vi "Получение данных.vi"(8 "error in (no error)":errorcluster, 11 "VISA Refnum in":refnum<visa-resource-name>) -> (0 "error out":errorcluster, 2 "String":string, 3 "VISA Refnum out":refnum<visa-resource-name>)   [LabVIEW 2013]
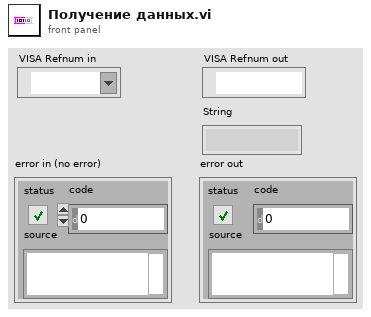
[diagram p1: front panel]
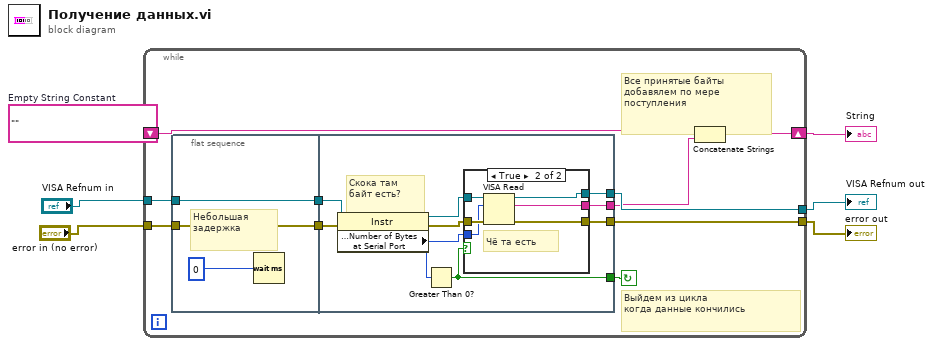
[diagram p0: block diagram]
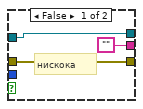
[diagram p2: hidden frame]
diagram:
  w1 = ""  # Empty String Constant
  n1 = while {
    tunnel: "VISA Refnum in" -> [w14]
    tunnel: "error in (no error)" -> [w13]
    tunnel: [w11] -> w2
    shift-right: [w8] -> w4
    shift-left: w1 -> [w10]
    tunnel: [w7] -> w3
    stop <- w12 continue-if-true
    # "Все принятые байты\nдобавялем по мере\nпоступления"
    # "Выйдем из цикла\nкогда данные кончились"
    n2 = flat-sequence {
      tunnel: w14 -> [w19]
      tunnel: w13 -> [w18]
      tunnel: [w19] -> w16
      tunnel: [w18] -> w15
      tunnel: w16 -> [w28]
      tunnel: w15 -> [w27]
      tunnel: [w23] -> w12
      tunnel: [w22] -> w9
      tunnel: [w21] -> w11
      tunnel: [w20] -> w7
      frame #0 {
        # "Небольшая\nзадержка"
        n3 = Wait (ms)(milliseconds to wait=u32 0) -> ()  [unwired: 1 out]
      }
      frame #1 {
        # "Скока там\nбайт есть?"
        n4 = property class="Instr"(reference=w28, error in=w27) -> (reference out=w26:refnum<visa-resource-name>, error out=w25:errorcluster, "Serial Settings:Number of Bytes at Serial Port"=w24:u32)
        n5 = Greater Than 0?(x=w24) -> (x > 0?=w23:bool)
        n6 = case shown="True" w23 {
          tunnel: w26 -> [w30 w37]
          tunnel: w25 -> [w31 w36]
          tunnel: w24 -> [_ w35]
          tunnel: [w31 w34] -> w20
          tunnel: [w30 w33] -> w21
          tunnel: ["" w32] -> w22
          frame False {
            # "нискока"
          }
          frame True {
            # "Чё та есть"
            n7 = VISA Read(VISA resource name=w37, byte count=w35, error in (no error)=w36) -> (VISA resource name out=w33:refnum<visa-resource-name>, read buffer=w32:string, error out=w34:errorcluster)  [unwired: 1 out]
          }
        }
      }
    }
    n8 = Concatenate Strings(w10, w9) -> (w8:string)
  }
  "String" <- w4
  "error out" <- w3
  "VISA Refnum out" <- w2
